vi "1A Helper - Init Sensor.vi"(8 "error in (no error)":errorcluster, 11 "VISA Refnum in":refnum<visa-resource-name>="COM1") -> (0 "error out":errorcluster, 2 "Try #":i32, 3 "VISA Refnum out":refnum<visa-resource-name>)   [LabVIEW 2011]
doc: "This VI checks to see if the sensor is communicating on 4800 or 38400 baud and sets it to 38400 baud if it is not already."
uses:
  2-Think/2 Typedefs/indicator LED.ctl
  2-Think/2 Globals/2 Global.vi
panel:
  out "# of serial connection attempts":i32
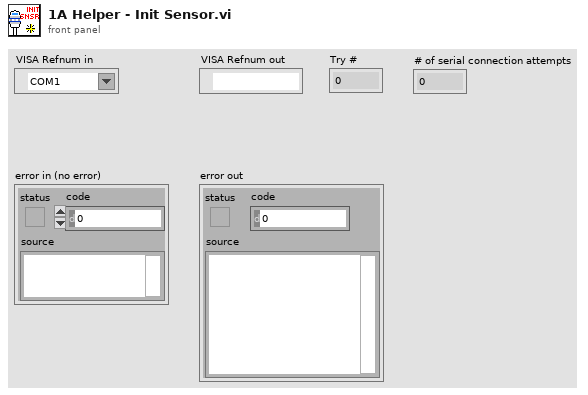
[diagram p1: front panel]
types:
  T1 = typedef "indicator LED.ctl" = bool
  T2 = typedef "generalized sensor status.ctl" = cluster{"Sensor Connected":T1, "Sensor Initialized":T1, "Sensor OK":T1, "Latest Error String":string, "GPS Lock":T1}
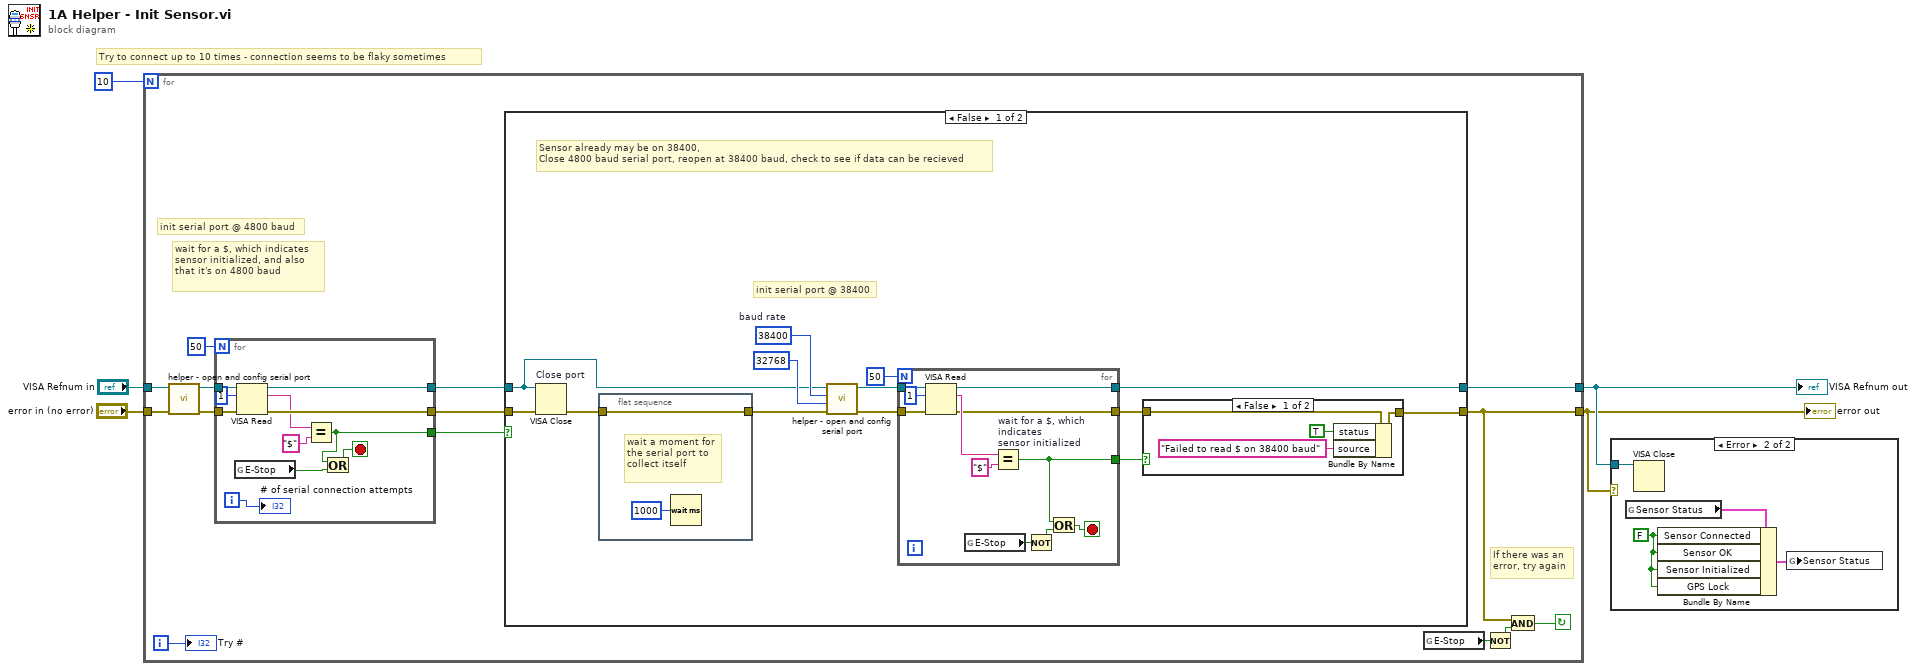
[diagram p0: block diagram]
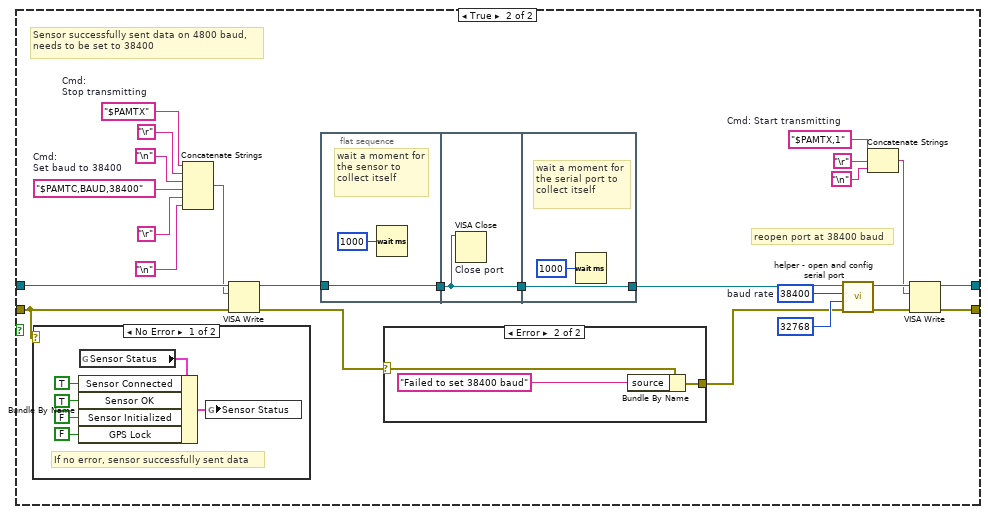
[diagram p3: hidden frame]
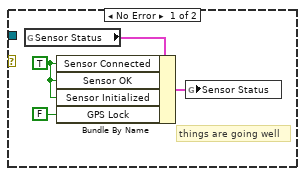
[diagram p6: hidden frame]
diagram:
  # "Try to connect up to 10 times - connection seems to be flaky sometimes"
  n1 = for {
    N: 10 -> [_]
    tunnel: "error in (no error)" -> [w19]
    tunnel: "VISA Refnum in" -> [w18]
    tunnel: [w17] -> w3
    tunnel: [w9] -> w2
    i -> [w11]
    stop <- w10 continue-if-true
    # "If there was an \nerror, try again"
    # "wait for a $, which indicates sensor initialized, and also that it's on 4800 baud"
    # "init serial port @ 4800 baud"
    n2 = call "helper - open and config serial port.vi"("error in (no error)"=w19, "VISA Refnum in"=w18) -> ("error out"=w14:errorcluster, "VISA Refnum out"=w15:refnum<visa-resource-name>)  [unwired: 8 in]
    n3 = for {
      N: 50 -> [_]
      tunnel: [w30] -> w16
      tunnel: w15 -> [w29]
      tunnel: w14 -> [w28]
      tunnel: [w27] -> w13
      tunnel: [w22] -> w12
      i -> [w21]
      stop <- w23 stop-if-true
      n4 = global read "2 Global.vi" "E-Stop"() -> (w20:bool)
      n5 = VISA Read(VISA resource name=w29, byte count=u32 1, error in (no error)=w28) -> (VISA resource name out=w30:refnum<visa-resource-name>, read buffer=w25:string, error out=w27:errorcluster)  [unwired: 1 out]
      n6 = Equal? ("wait for a $, which indicates\nsensor initialized")(x=w25, y="$" ("x")) -> (x = y?=w22:bool)
      n7 = Or(x=w22, y=w20) -> (x .or. y?=w23:bool)
      "# of serial connection attempts" <- w21
    }
    n8 = case shown="False" w12 {
      tunnel: [w39 w82] -> w17
      tunnel: w16 -> [w31 w74]
      tunnel: w13 -> [w34 w64]
      tunnel: [w38 w69] -> w9
      frame False {
        w43 = u32 38400  # baud rate
        # "init serial port @ 38400"
        # "Sensor already may be on 38400,\nClose 4800 baud serial port, reopen at 38400 baud, check to see if data can be recieved"
        n9 = VISA Close "Close port"(VISA resource name=w31, error in (no error)=w34) -> (error out=w33:errorcluster)
        n10 = flat-sequence {
          tunnel: w33 -> [w44]
          tunnel: [w44] -> w32
          frame #0 {
            # "wait a moment for the serial port to collect itself"
            n11 = Wait (ms)(milliseconds to wait=u32 1000) -> ()  [unwired: 1 out]
          }
        }
        n12 = call "helper - open and config serial port.vi"("error in (no error)"=w32, "Input\nbuffer size"=u32 32768 ("Input\nbuffer size"), "baud rate"=w43, "VISA Refnum in"=w31) -> ("error out"=w40:errorcluster, "VISA Refnum out"=w41:refnum<visa-resource-name>)  [unwired: 6 in]
        n13 = for {
          N: 50 -> [_]
          tunnel: w41 -> [w56]
          tunnel: w40 -> [w55]
          tunnel: [w54] -> w39
          tunnel: [w46] -> w37
          tunnel: [w50] -> w36
          stop <- w47 stop-if-true
          n14 = VISA Read(VISA resource name=w56, byte count=u32 1, error in (no error)=w55) -> (VISA resource name out=w54:refnum<visa-resource-name>, read buffer=w52:string, error out=w50:errorcluster)  [unwired: 1 out]
          n15 = global read "2 Global.vi" "E-Stop"() -> (w48:bool)
          n16 = Equal? "wait for a $, which indicates\nsensor initialized"(x=w52, y="$" ("x")) -> (x = y?=w46:bool)
          n17 = Not(x=w48) -> (.not. x?=w49:bool)
          n18 = Or(x=w46, y=w49) -> (x .or. y?=w47:bool)
        }
        n19 = case shown="False" w37 {
          tunnel: w36 -> [w58 w61]
          tunnel: [w57 w61] -> w38
          frame False {
            n20 = Bundle By Name(cluster=w58, "status"=TRUE, "source"="Failed to read $ on 38400 baud") -> (w57:errorcluster)
          }
          frame True {
          }
        }
      }
      frame True {
        w68 = "$PAMTC,BAUD,38400"  # Cmd: Set baud to 38400
        w73 = "$PAMTX"  # Cmd: Stop transmitting
        w78 = "$PAMTX,1"  # Cmd: Start transmitting
        w84 = u32 38400  # baud rate
        # "Sensor successfully sent data on 4800 baud,\nneeds to be set to 38400"
        # "reopen port at 38400 baud"
        n21 = case shown="No Error" w64 {
          frame No Error {
            # "If no error, sensor successfully sent data"
            n22 = global read "2 Global.vi" "Sensor Status"() -> (w95:T2)
            n23 = Bundle By Name(cluster=w95, "Sensor Connected"=T1 TRUE, "Sensor OK"=T1 TRUE, "Sensor Initialized"=T1 FALSE, "GPS Lock"=T1 FALSE) -> (w96:T2)
            n24 = global write "2 Global.vi" "Sensor Status"(w96) -> ()
          }
          frame Error {
          }
        }
        n25 = Concatenate Strings(w73, "\r" ("Carriage Return Constant"), "\n", w68, "\r" ("Carriage Return Constant"), "\n") -> (w72:string)
        n26 = VISA Write(VISA resource name=w74, write buffer=w72, error in (no error)=w64) -> (VISA resource name out=w65:refnum<visa-resource-name>, error out=w63:errorcluster)  [unwired: 1 out]
        n27 = flat-sequence {
          tunnel: w65 -> [w97]
          tunnel: [w97] -> w86
          tunnel: w86 -> [w99]
          tunnel: [w99] -> w85
          tunnel: [w101] -> w83
          tunnel: w85 -> [w101]
          frame #0 {
            # "wait a moment for the sensor to collect itself"
            n28 = Wait (ms)(milliseconds to wait=u32 1000) -> ()  [unwired: 1 out]
          }
          frame #1 {
            n29 = VISA Close "Close port"(VISA resource name=w99) -> ()  [unwired: 1 in, 1 out]
          }
          frame #2 {
            # "wait a moment for the serial port to collect itself"
            n30 = Wait (ms)(milliseconds to wait=u32 1000) -> ()  [unwired: 1 out]
          }
        }
        n31 = case shown="Error" w63 {
          selector: w63 -> [w87 w90]
          tunnel: [w87 w88] -> w62
          frame No Error {
          }
          frame Error {
            n32 = Bundle By Name(cluster=w90, "source"="Failed to set 38400 baud") -> (w88:errorcluster)
          }
        }
        n33 = call "helper - open and config serial port.vi"("error in (no error)"=w62, "Input\nbuffer size"=u32 32768 ("Input\nbuffer size"), "baud rate"=w84, "VISA Refnum in"=w83) -> ("error out"=w81:errorcluster, "VISA Refnum out"=w79:refnum<visa-resource-name>)  [unwired: 6 in]
        n34 = Concatenate Strings(w78, "\r" ("Carriage Return Constant"), "\n") -> (w75:string)
        n35 = VISA Write(VISA resource name=w79, write buffer=w75, error in (no error)=w81) -> (VISA resource name out=w82:refnum<visa-resource-name>, error out=w69:errorcluster)  [unwired: 1 out]
      }
    }
    n36 = global read "2 Global.vi" "E-Stop"() -> (w7:bool)
    n37 = Not(x=w7) -> (.not. x?=w8:bool)
    n38 = And(x=w9, y=w8) -> (x .and. y?=w10:bool)
    "Try #" <- w11
  }
  "VISA Refnum out" <- w3
  "error out" <- w2
  n39 = case shown="Error" w2 {
    tunnel: w3 -> [_ w109]
    frame No Error {
      w103 = T1 TRUE ("Sensor Connected")
      # "things are going well"
      n40 = global read "2 Global.vi" "Sensor Status"() -> (w104:T2)
      n41 = Bundle By Name(cluster=w104, "Sensor Connected"=w103, "Sensor OK"=w103, "Sensor Initialized"=w103, "GPS Lock"=T1 FALSE) -> (w105:T2)
      n42 = global write "2 Global.vi" "Sensor Status"(w105) -> ()
    }
    frame Error {
      w106 = T1 FALSE ("Sensor Connected")
      n43 = global read "2 Global.vi" "Sensor Status"() -> (w107:T2)
      n44 = VISA Close(VISA resource name=w109) -> ()  [unwired: 1 in, 1 out]
      n45 = Bundle By Name(cluster=w107, "Sensor Connected"=w106, "Sensor OK"=w106, "Sensor Initialized"=w106, "GPS Lock"=w106) -> (w108:T2)
      n46 = global write "2 Global.vi" "Sensor Status"(w108) -> ()
    }
  }
